vi "configureDDSOutput.vi"(8 "error in (no error)":errorcluster, 9 "DDSOutput":refnum<class "DDSOutput.lvclass">, 10 "device":string, 11 "AtomChipHWC in":refnum<class "AtomChipHWC.lvclass">) -> (0 "error out":errorcluster, 3 "AtomChipHWC out":refnum<class "AtomChipHWC.lvclass">)   [LabVIEW 2011, in "Hardware.lvlib" / "HWControllers.lvlib" / "AtomChipHWC.lvclass"]
uses:
  AtomChipHWC.lvclass
  Channels/DDSOutput/Generic/DDSOutput.lvclass
  AtomChipHWC.lvclass/AtomChipHWC.ctl
  HWController.lvclass
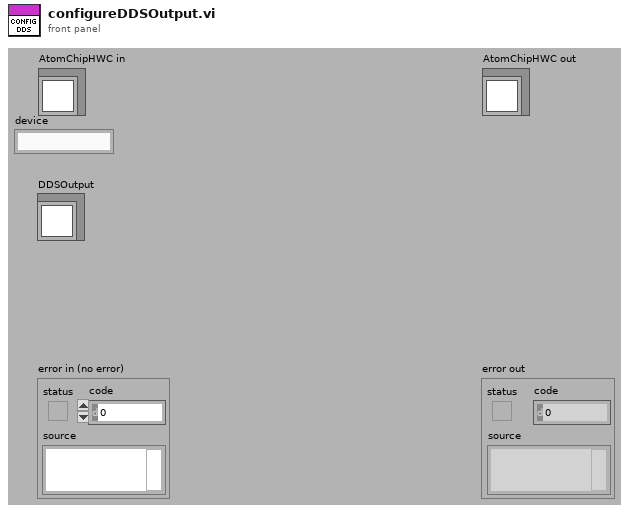
[diagram p1: front panel]
types:
  T1 = cluster{"OutputForm":enum16{"Sine", "Square", "Triangle", "Arbitrary"}[], "OutputFunction":enum16{"Frequency", "Ramp", "Sequence"}[], "physicalChannels":string}
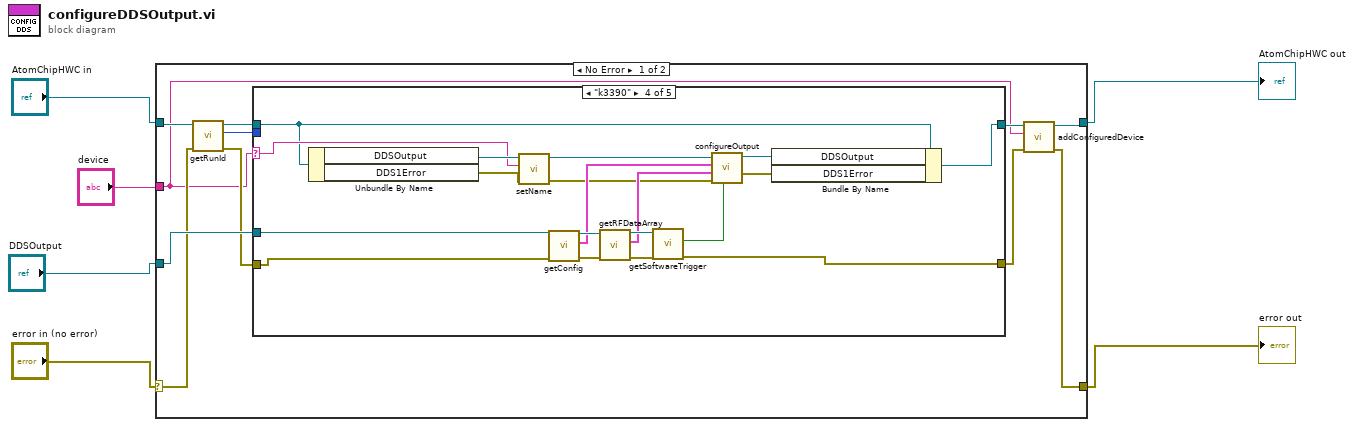
[diagram p0: block diagram]
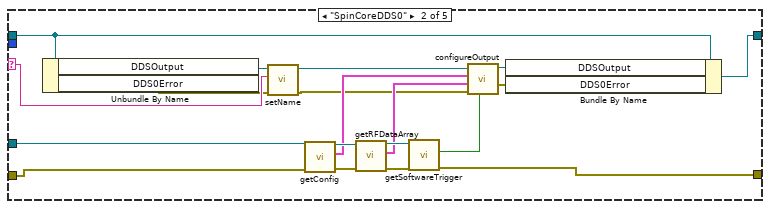
[diagram p3: hidden frame]
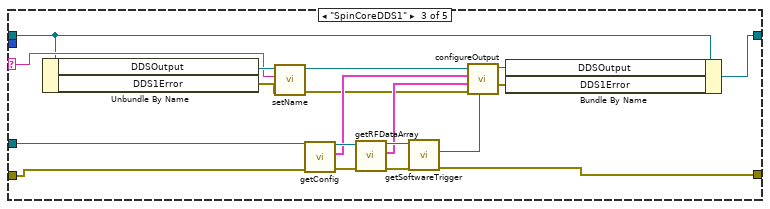
[diagram p4: hidden frame]
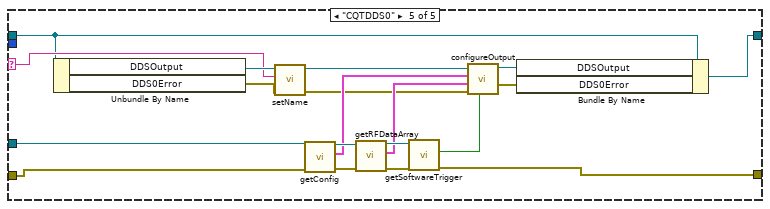
[diagram p5: hidden frame]
diagram:
  n1 = case shown="No Error" "error in (no error)" {
    selector: "error in (no error)" -> [w10 w97]
    tunnel: [w13 w97] -> w3
    tunnel: [w15 w96] -> w4
    tunnel: "AtomChipHWC in" -> [w11 w96]
    tunnel: "device" -> [w7 _]
    tunnel: "DDSOutput" -> [w17 _]
    frame No Error {
      n2 = call "getRunId.vi"("error in (no error)"=w10, "HWController in"=w11) -> ("error out"=w9:errorcluster, "Numeric"=w8:i32, "HWController out"=w12:refnum<class "AtomChipHWC.lvclass">)  [unwired: 7 in]
      n3 = case shown="\"k3390\"" w7 {
        selector: w7 -> [_ w37 w56 w75 w94]
        tunnel: w12 -> [w19 w29 w48 w67 w86]
        tunnel: [w19 w25 w44 w63 w82] -> w16
        tunnel: [w18 w20 w40 w59 w78] -> w14
        tunnel: w17 -> [_ w27 w46 w65 w84]
        tunnel: w9 -> [w18 w21 w39 w58 w77]
        tunnel: w8 -> [_ _ _ _ _]
        frame "No Hardware", Default {
        }
        frame "SpinCoreDDS0" {
          n4 = Unbundle By Name(w29) -> ("DDSOutput"=w38:refnum<class "DDSOutput.lvclass">, "DDS0Error"=w24:errorcluster)
          n5 = call "setName.vi"("error in (no error)"=w24, "name"=w37, "DDSOutput in"=w38) -> ("error out"=w22:errorcluster, "DDSOutput out"=w34:refnum<class "DDSOutput.lvclass">)  [unwired: 7 in]
          n6 = call "getConfig.vi"("error in (no error)"=w21, "DDSOutput in"=w27) -> ("error out"=w30:errorcluster, "Config"=w26:T1, "DDSOutput out"=w31:refnum<class "DDSOutput.lvclass">)  [unwired: 7 in]
          n7 = call "getRFDataArray.vi"("error in (no error)"=w30, "DDSOutput in"=w31) -> ("error out"=w35:errorcluster, "rfDataArray"=w33:cluster{dbl[][]}[], "DDSOutput out"=w36:refnum<class "DDSOutput.lvclass">)  [unwired: 7 in]
          n8 = call "getSoftwareTrigger.vi"("error in (no error)"=w35, "DDSOutput in"=w36) -> ("error out"=w20:errorcluster, "softwareTrigger"=w32:bool)  [unwired: 7 in, 1 out]
          n9 = call-dynamic "configureOutput.vi"("sofwareTrigger?"=w32, "error in (no error)"=w22, "Data"=w33, "Config"=w26, "DDSOutput in"=w34) -> ("error out"=w23:errorcluster, "DDSOutput out"=w28:refnum<class "DDSOutput.lvclass">)  [unwired: 5 in]
          n10 = Bundle By Name(cluster=w29, "DDSOutput"=w28, "DDS0Error"=w23) -> (w25:refnum<class "AtomChipHWC.lvclass">)
        }
        frame "SpinCoreDDS1" {
          n11 = Unbundle By Name(w48) -> ("DDSOutput"=w57:refnum<class "DDSOutput.lvclass">, "DDS1Error"=w43:errorcluster)
          n12 = call "setName.vi"("error in (no error)"=w43, "name"=w56, "DDSOutput in"=w57) -> ("error out"=w42:errorcluster, "DDSOutput out"=w53:refnum<class "DDSOutput.lvclass">)  [unwired: 7 in]
          n13 = call "getConfig.vi"("error in (no error)"=w39, "DDSOutput in"=w46) -> ("error out"=w49:errorcluster, "Config"=w45:T1, "DDSOutput out"=w50:refnum<class "DDSOutput.lvclass">)  [unwired: 7 in]
          n14 = call "getRFDataArray.vi"("error in (no error)"=w49, "DDSOutput in"=w50) -> ("error out"=w54:errorcluster, "rfDataArray"=w52:cluster{dbl[][]}[], "DDSOutput out"=w55:refnum<class "DDSOutput.lvclass">)  [unwired: 7 in]
          n15 = call "getSoftwareTrigger.vi"("error in (no error)"=w54, "DDSOutput in"=w55) -> ("error out"=w40:errorcluster, "softwareTrigger"=w51:bool)  [unwired: 7 in, 1 out]
          n16 = call-dynamic "configureOutput.vi"("sofwareTrigger?"=w51, "error in (no error)"=w42, "Data"=w52, "Config"=w45, "DDSOutput in"=w53) -> ("error out"=w41:errorcluster, "DDSOutput out"=w47:refnum<class "DDSOutput.lvclass">)  [unwired: 5 in]
          n17 = Bundle By Name(cluster=w48, "DDSOutput"=w47, "DDS1Error"=w41) -> (w44:refnum<class "AtomChipHWC.lvclass">)
        }
        frame "k3390" {
          n18 = Unbundle By Name(w67) -> ("DDSOutput"=w76:refnum<class "DDSOutput.lvclass">, "DDS1Error"=w62:errorcluster)
          n19 = call "setName.vi"("error in (no error)"=w62, "name"=w75, "DDSOutput in"=w76) -> ("error out"=w61:errorcluster, "DDSOutput out"=w72:refnum<class "DDSOutput.lvclass">)  [unwired: 7 in]
          n20 = call "getConfig.vi"("error in (no error)"=w58, "DDSOutput in"=w65) -> ("error out"=w68:errorcluster, "Config"=w64:T1, "DDSOutput out"=w69:refnum<class "DDSOutput.lvclass">)  [unwired: 7 in]
          n21 = call "getRFDataArray.vi"("error in (no error)"=w68, "DDSOutput in"=w69) -> ("error out"=w73:errorcluster, "rfDataArray"=w71:cluster{dbl[][]}[], "DDSOutput out"=w74:refnum<class "DDSOutput.lvclass">)  [unwired: 7 in]
          n22 = call "getSoftwareTrigger.vi"("error in (no error)"=w73, "DDSOutput in"=w74) -> ("error out"=w59:errorcluster, "softwareTrigger"=w70:bool)  [unwired: 7 in, 1 out]
          n23 = call-dynamic "configureOutput.vi"("sofwareTrigger?"=w70, "error in (no error)"=w61, "Data"=w71, "Config"=w64, "DDSOutput in"=w72) -> ("error out"=w60:errorcluster, "DDSOutput out"=w66:refnum<class "DDSOutput.lvclass">)  [unwired: 5 in]
          n24 = Bundle By Name(cluster=w67, "DDSOutput"=w66, "DDS1Error"=w60) -> (w63:refnum<class "AtomChipHWC.lvclass">)
        }
        frame "CQTDDS0" {
          n25 = Unbundle By Name(w86) -> ("DDSOutput"=w95:refnum<class "DDSOutput.lvclass">, "DDS0Error"=w81:errorcluster)
          n26 = call "setName.vi"("error in (no error)"=w81, "name"=w94, "DDSOutput in"=w95) -> ("error out"=w80:errorcluster, "DDSOutput out"=w91:refnum<class "DDSOutput.lvclass">)  [unwired: 7 in]
          n27 = call "getConfig.vi"("error in (no error)"=w77, "DDSOutput in"=w84) -> ("error out"=w87:errorcluster, "Config"=w83:T1, "DDSOutput out"=w88:refnum<class "DDSOutput.lvclass">)  [unwired: 7 in]
          n28 = call "getRFDataArray.vi"("error in (no error)"=w87, "DDSOutput in"=w88) -> ("error out"=w92:errorcluster, "rfDataArray"=w90:cluster{dbl[][]}[], "DDSOutput out"=w93:refnum<class "DDSOutput.lvclass">)  [unwired: 7 in]
          n29 = call "getSoftwareTrigger.vi"("error in (no error)"=w92, "DDSOutput in"=w93) -> ("error out"=w78:errorcluster, "softwareTrigger"=w89:bool)  [unwired: 7 in, 1 out]
          n30 = call-dynamic "configureOutput.vi"("sofwareTrigger?"=w89, "error in (no error)"=w80, "Data"=w90, "Config"=w83, "DDSOutput in"=w91) -> ("error out"=w79:errorcluster, "DDSOutput out"=w85:refnum<class "DDSOutput.lvclass">)  [unwired: 5 in]
          n31 = Bundle By Name(cluster=w86, "DDSOutput"=w85, "DDS0Error"=w79) -> (w82:refnum<class "AtomChipHWC.lvclass">)
        }
      }
      n32 = call "addConfiguredDevice.vi"("error in (no error)"=w14, "deviceName"=w7, "HWController in"=w16) -> ("error out"=w13:errorcluster, "HWController out"=w15:refnum<class "AtomChipHWC.lvclass">)  [unwired: 7 in]
    }
    frame Error {
    }
  }
  "error out" <- w3
  "AtomChipHWC out" <- w4
